vi "Test_2.vi"(10 "y":dbl, 11 "Slide":dbl) -> (3 "Gauge":dbl(knob) scale=0.0..15.0)   [LabVIEW 2015]
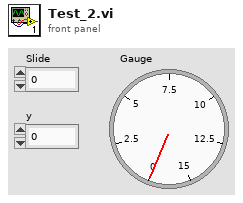
[diagram p1: front panel]
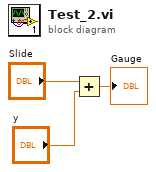
[diagram p0: block diagram]
diagram:
  n1 = Add(x="Slide", y="y") -> (x+y=→"Gauge":dbl)
